vi "数值控件的属性.vi"() -> ()   [LabVIEW 2013]
panel:
  in  "滚动条":i32(c297)
  out "量表":cluster{dbl, dbl}(knob) scale=0.0..10.0
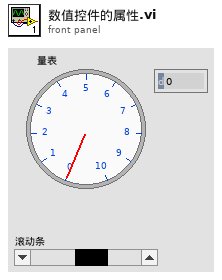
[diagram p1: front panel]
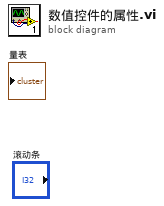
[diagram p0: block diagram]
diagram:
